vi "Send Write Record.vi"(7 "Message Priority (Normal)":T3=enum."Normal", 8 "error in (no error)":errorcluster, 10 "Record":T1 {"Step Duration" format="%_5g"}, 11 "Message Enqueuer":refnum<class "Message Enqueuer.lvclass">) -> (0 "error out":errorcluster, 3 "Message Enqueuer out":refnum<class "Message Enqueuer.lvclass">)   [LabVIEW 2019, in "Sim Configuration Database Actor.lvlib" / "Write Record Msg.lvclass"]
doc: "This VI sends the message to an actor."
uses:
  Write Record Msg.lvclass
  <vilib>/ActorFramework/Message Enqueuer/Message Enqueuer.lvclass
  <vilib>/ActorFramework/Message Enqueuer/Message Priority.ctl
  Sim Configuration Database Actor/Record.ctl
  Vehicle Position Simulation Actor/Car Wash Controller/Station -Enum.ctl
  C:/Program Files (x86)/National Instruments/LabVIEW 2019/vi.lib/ActorFramework/Message/Message.lvclass
  Write Record Msg.lvclass/Write Record Msg.ctl
  <vilib>/ActorFramework/Message Enqueuer/Message Enqueuer.lvclass/Message Enqueuer.ctl
  <vilib>/ActorFramework/Message Priority Queue/Priority Enqueue.vi
  Sim Configuration Database Actor/Sim Configuration Database Actor.lvclass
  Vehicle Position Simulation Actor/Car Wash Controller/Vehicle Position Simulation Actor.lvclass
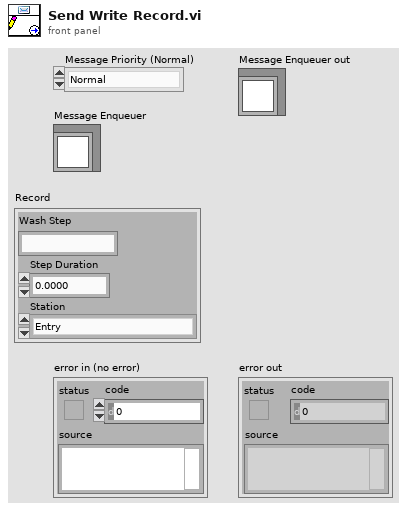
[diagram p1: front panel]
types:
  T1 = typedef "Sim Configuration Database Actor.lvlib/Sim Configuration Database Actor.lvclass/Record.ctl" = cluster{"Wash Step":string, "Step Duration":dbl, "Station":T2}
  T2 = typedef "Vehicle Position Sinmulation Actor.lvlib/Vehicle Position Simulation Actor.lvclass/Station -Enum.ctl" = enum16{"Entry", "Station1", "Station2", "Station3", "Exit"}
  T3 = typedef "Actor Framework.lvlib/Message Enqueuer.lvclass/Message Priority.ctl" = enum16{"Low", "Normal", "High"}
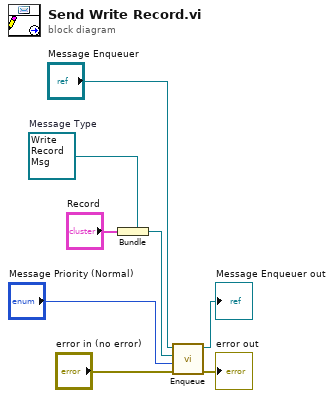
[diagram p0: block diagram]
diagram:
  w5 = refnum<class "Write Record Msg.lvclass"> refnum  # Message Type
  n1 = Bundle(cluster=w5, "Record") -> (w4:refnum<class "Write Record Msg.lvclass">)
  n2 = call <vilib>:"Enqueue.vi"("error in (no error)"="error in (no error)", "Message Priority (Normal)"="Message Priority (Normal)", "Message"=w4, "Message Enqueuer in"="Message Enqueuer") -> ("error out"=→"error out":errorcluster, "Message Enqueuer out"=→"Message Enqueuer out":refnum<class "Message Enqueuer.lvclass">)  [unwired: 6 in]
